vi "DHE_DRV_set_geom.vi"(0 "fd":i32, 1 "ypredata":i32, 2 "ypostdata":i32, 5 "xpredata":i32, 7 "xpostdata":i32, 9 "xdata":i32, 11 "error in (no error)":errorcluster, 12 "ydata":i32) -> (4 "fd out":i32, 8 "return value":i32, 15 "error out":errorcluster)   [LabVIEW 2016]
doc: "This VI closes the I/O interface with the instrument."
uses:
  c/lib/libarcDHE.so
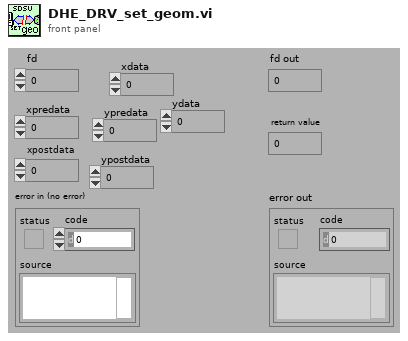
[diagram p1: front panel]
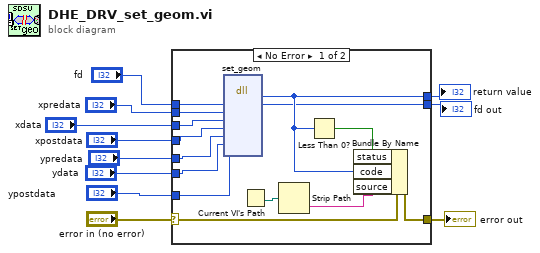
[diagram p0: block diagram]
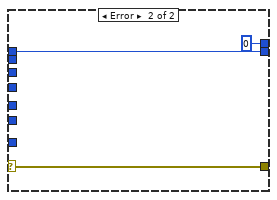
[diagram p2: hidden frame]
diagram:
  n1 = case shown="No Error" "error in (no error)" {
    selector: "error in (no error)" -> [w17 w26]
    tunnel: "fd" -> [w25 w28]
    tunnel: [w23 0] -> w10
    tunnel: [w20 w26] -> w9
    tunnel: "xpredata" -> [w19 _]
    tunnel: "xpostdata" -> [w15 _]
    tunnel: [w18 w28] -> w6
    tunnel: "ypredata" -> [w14 _]
    tunnel: "ypostdata" -> [w12 _]
    tunnel: "ydata" -> [w13 _]
    tunnel: "xdata" -> [w16 _]
    frame No Error {
      n2 = dll-call lib="home/simager/panview/PAN/Modules/SDSU/private/c/lib/libarcDHE.so" fn="set_geom"("fd"=w25, "xpre"=w19, "xdata"=w16, "xov"=w15, "ypre"=w14, "ydata"=w13, "yov"=w12) -> (w23:i32, "fd"=w18:i32)  [unwired: 9 in, 2 out]
      n3 = Current VI's Path() -> (path=w22:path)
      n4 = Strip Path(path=w22) -> (name=w21:string)  [unwired: 1 out]
      n5 = Less Than 0?(x=w23) -> (x < 0?=w24:bool)
      n6 = Bundle By Name(cluster=w17, "status"=w24, "code"=w23, "source"=w21) -> (w20:errorcluster)
    }
    frame Error {
    }
  }
  "error out" <- w9
  "return value" <- w10
  "fd out" <- w6
